vi "PJVS waveform.vi"() -> ()   [LabVIEW 2020]
uses:
  Public/Configure/Configure Waveform (Arbitrary).vi
  Keithley 3390.lvlib
panel:
  in  "upload":bool caption="Check to upload waveform to AWG"
  out "Coherent?":bool
  out "PJVS segment\nvoltages (V)":dbl[](array[numeric])
  out "Length of segment (samples)":dbl format="%.3g"
  in  "PJVS segments":i32=20 min=2 step=1
  out "Waveform Graph":dbl[](graph)
  in  "Timeout for upload to the AWG (ms)":u32=30000 min=1000 step=1
  in  "Samples":i32=10000 min=10 max=256000 step=1
  in  "Sine amplitude (V)":dbl=1.0 min=-10.1 max=10.1 format="%#_13g"
  in  "Offset (V)":dbl
  in  "Frequency (Hz)":dbl=50.0
  in  "Arbitrary Waveform Name":string="PJVS1"
  in  "AWG VISA resource name":refnum<visa-resource-name>
  # "For large waveform transfers, increase the timeout value."
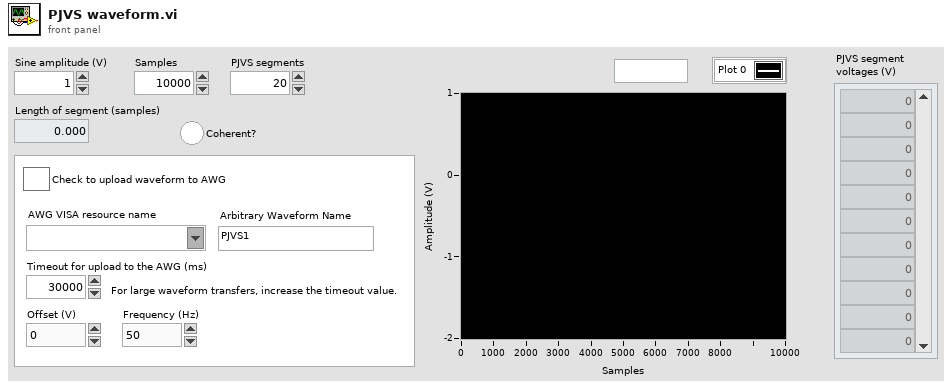
[diagram p1: front panel]
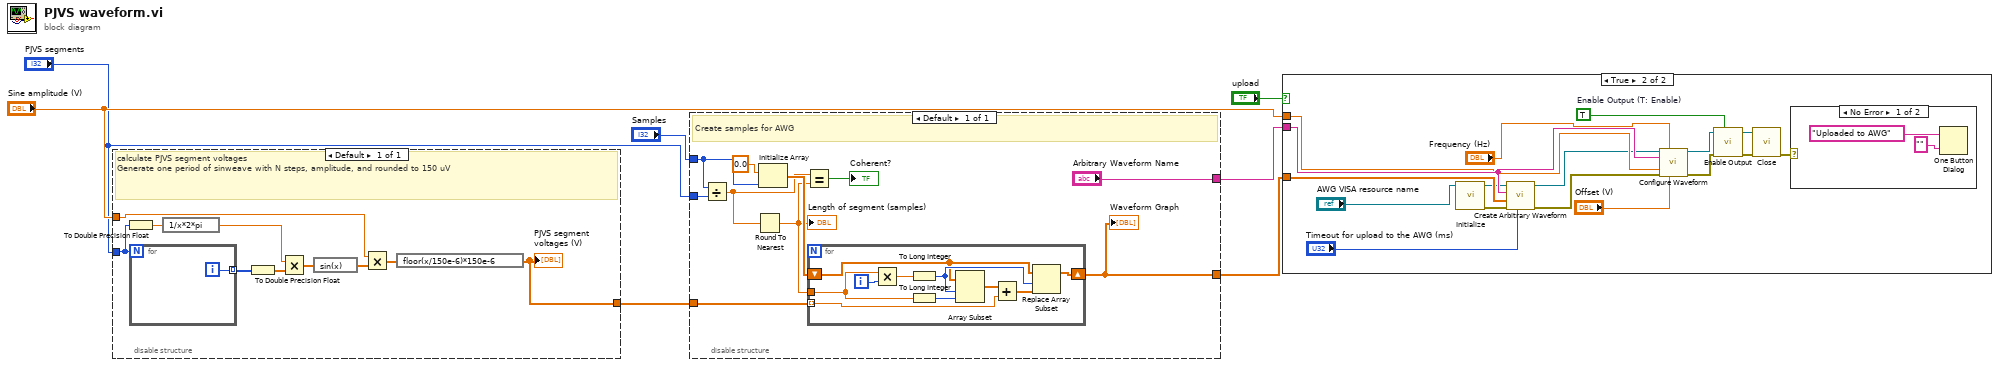
[diagram p0: block diagram]
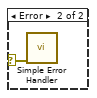
[diagram p3: hidden frame]
diagram:
  n1 = disable-structure shown="Default" {
    disable-tunnel: "Sine amplitude (V)" -> [w11]
    disable-tunnel: "PJVS segments" -> [w10]
    disable-tunnel: [w8] -> w5
    frame Enabled {
      # "calculate PJVS segment voltages\nGenerate one period of sinweave with N steps, amplitude, and rounded to 150 uV"
      n2 = To Double Precision Float(number=w10) -> (double precision float=w17:dbl)
      n3 = for {
        N: w10 -> [_]
        tunnel: [w18] -> w15 mode=indexing
        i -> [w18]
      }
      n4 = expression code="1/x*2*pi"(w17) -> (w14:dbl)
      n5 = To Double Precision Float(number=w15) -> (double precision float=w16:dbl[])
      n6 = Multiply(x=w14, y=w16) -> (x*y=w13:dbl[])
      n7 = expression code="sin(x)"(w13) -> (w12:dbl[])
      n8 = Multiply(x=w11, y=w12) -> (x*y=w9:dbl[])
      n9 = expression code="floor(x/150e-6)*150e-6"(w9) -> (w8:dbl[])
      "PJVS segment\nvoltages (V)" <- w8
    }
  }
  n10 = disable-structure shown="Default" {
    disable-tunnel: ["Arbitrary Waveform Name"] -> w7
    disable-tunnel: w5 -> [w27]
    disable-tunnel: "PJVS segments" -> [w26]
    disable-tunnel: [w25] -> w3
    disable-tunnel: "Samples" -> [w23]
    frame Enabled {
      # "Create samples for AWG"
      n11 = Divide(x=w23, y=w26) -> (x/y=w21:dbl)
      n12 = Round To Nearest(number=w21) -> (nearest integer value=w20:dbl)
      "Length of segment (samples)" <- w20
      n13 = Initialize Array(0.0 ("element"), w23) -> (w22:dbl[])
      n14 = Equal?(x=w21, y=w20) -> (x = y?=→"Coherent?":bool)
      n15 = for {
        tunnel: w27 -> [w32] mode=indexing
        shift-right: [w34] -> w25
        shift-left: w22 -> [w31]
        tunnel: w20 -> [w29]
        i -> [w38]
        n16 = Multiply(x=w29, y=w38) -> (x*y=w36:dbl)
        n17 = To Long Integer(number=w36) -> (32bit integer=w35:i32)
        n18 = To Long Integer(number=w29) -> (32bit integer=w37:i32)
        n19 = Array Subset(array=w31, index=w35, length=w37) -> (w33:dbl[])
        n20 = Add(x=w33, y=w32) -> (x+y=w30:dbl[])
        n21 = Replace Array Subset(array=w31, new element=w30, index=w35) -> (w34:dbl[])
      }
      "Waveform Graph" <- w25
    }
  }
  n22 = case shown="True" "upload" {
    tunnel: w7 -> [_ w55]
    tunnel: "Sine amplitude (V)" -> [_ w54]
    tunnel: w3 -> [_ w53]
    frame False {
    }
    frame True {
      w47 = TRUE  # Enable Output (T: Enable)
      n23 = call "Initialize.vi"("VISA resource name"="AWG VISA resource name") -> ("error out"=w49:errorcluster, "VISA resource name out"=w48:refnum<visa-resource-name>)  [unwired: 9 in]
      n24 = call "Create Arbitrary Waveform.vi"("Timeout (10000 ms)"="Timeout for upload to the AWG (ms)", "error in (no error)"=w49, "Arbitrary Waveform Data"=w53, "Arbitrary Waveform Name (\"ARB1\")"=w55, "VISA resource name"=w48) -> ("error out"=w45:errorcluster, "VISA resource name out"=w44:refnum<visa-resource-name>)  [unwired: 5 in]
      n25 = call-poly "Configure Waveform.vi"("VISA resource name"=w44, "Frequency (1000 Hz)"="Frequency (Hz)", "Arbitrary Waveform Name (\"EXP_RISE\")"=w55, "Gain (1.0 Vpp)"=w54, "error in (no error)"=w45, "DC Offset (0.00 V)"="Offset (V)") -> ("VISA resource name out"=w43:refnum<visa-resource-name>, "error out"=w46:errorcluster)  [unwired: 8 in]
      n26 = call "Enable Output.vi"("Enable Output (T: Enable)"=w47, "error in (no error)"=w46, "VISA resource name"=w43) -> ("error out"=w51:errorcluster, "VISA resource name out"=w50:refnum<visa-resource-name>)  [unwired: 7 in]
      n27 = call "Close.vi"("error in (no error)"=w51, "VISA resource name"=w50) -> ("error out"=w39:errorcluster)  [unwired: 9 in]
      n28 = case shown="No Error" w39 {
        selector: w39 -> [_ w58]
        frame No Error {
          n29 = One Button Dialog(message="Uploaded to AWG", button name ("OK")="") -> ()  [unwired: 1 out]
        }
        frame Error {
          n30 = call <vilib>:"Simple Error Handler.vi"("error in (no error)"=w58) -> ()  [unwired: 4 in, 5 out]
        }
      }
    }
  }
